vi "游标显示-步响应.vi"(3 "步响应计算参数 in":T2, 4 "试验模式":string, 5 "reference in":refnum<vi>) -> (0 "步响应计算参数 out":T2, 1 "试验模式 out":string, 2 "reference out":refnum<vi>)   [LabVIEW 2013]
panel:
  in  "Array":string[](array[string])=["行程", "油压1"]
  out "Yrange":dbl
  out "Xrange":dbl
  in  "Cursor":T1
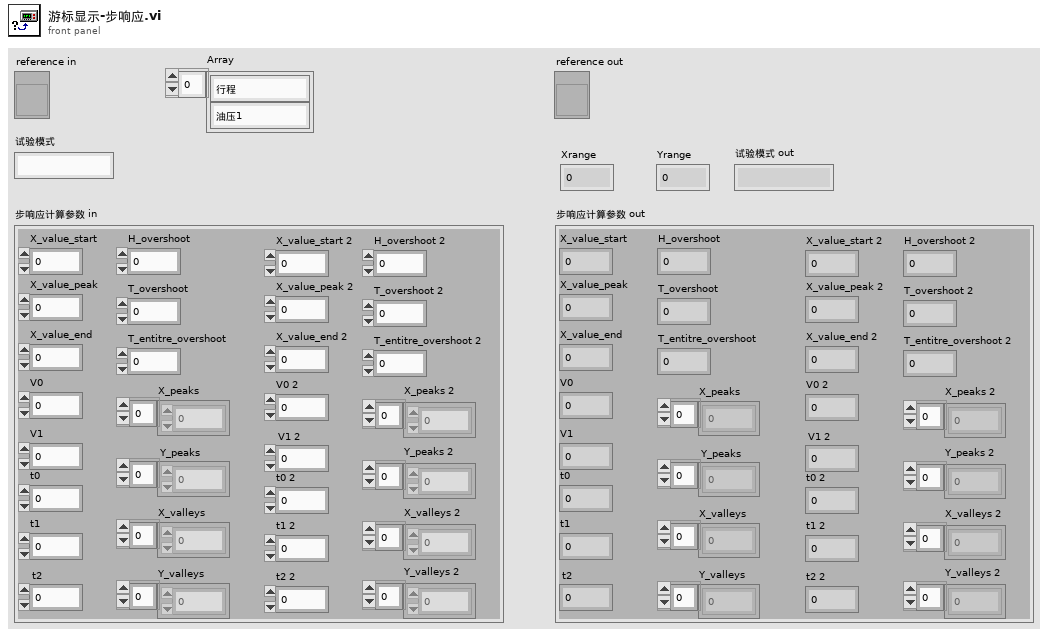
[diagram p1: front panel]
types:
  T1 = cluster{"Name":string, "Color":u32, "Style":u8, "Point Style":u8, "Name Visible":bool, "Allow Drag":bool, "Cursor Mode":u32, "Plot":i32, "Index":i32, "Position":cluster{"X":dbl, "Y":dbl}, "X Scale":u32, "Y Scale":u32, "Watch Plots":i32[], "Watch All Plots":bool, "Plot Area":i32, "Label Offset":cluster{"X":dbl, "Y":dbl}}
  T2 = cluster{"X_value_start":dbl, "X_value_peak":dbl, "t1":dbl, "X_value_end":dbl, "V0":dbl, "V1":dbl, "t0":dbl, "X_peaks":dbl[], "X_valleys":dbl[], "Y_peaks":dbl[], "Y_valleys":dbl[], "t2":dbl, "H_overshoot":dbl, "T_overshoot":dbl, "T_entitre_overshoot":dbl, "X_value_start 2":dbl, "X_value_peak 2":dbl, "t1 2":dbl, "X_value_end 2":dbl, "V0 2":dbl, "V1 2":dbl, "t0 2":dbl, "X_peaks 2":dbl[], "X_valleys 2":dbl[], "Y_peaks 2":dbl[], "t2 2":dbl, "H_overshoot 2":dbl, "T_overshoot 2":dbl, "T_entitre_overshoot 2":dbl, "Y_valleys 2":dbl[]}
  T3 = cluster{"Name":string, "Color":u32, "Style":u8, "Point Style":u8, "Name Visible":bool, "Allow Drag":bool, "Cursor Mode":u32, "Plot":i32, "Index":i32, "Position":cluster{"X":dbl, "Y":dbl}, "X Scale":u32, "Y Scale":u32, "Watch Plots":i32[], "Watch All Plots":bool, "Plot Area":i32, "Label Offset":cluster{"X":dbl, "Y":dbl}}[]
  T4 = typedef "LVCursorListTypeDef.ctl" = cluster{"Name":string, "Color":u32, "Style":u8, "Point Style":u8, "Name Visible":bool, "Allow Drag":bool, "Cursor Mode":u32, "Plot":i32, "Index":i32, "Position":cluster{"X":dbl, "Y":dbl}, "X Scale":u32, "Y Scale":u32, "Watch Plots":i32[], "Watch All Plots":bool, "Plot Area":i32, "Label Offset":cluster{"X":dbl, "Y":dbl}}[]
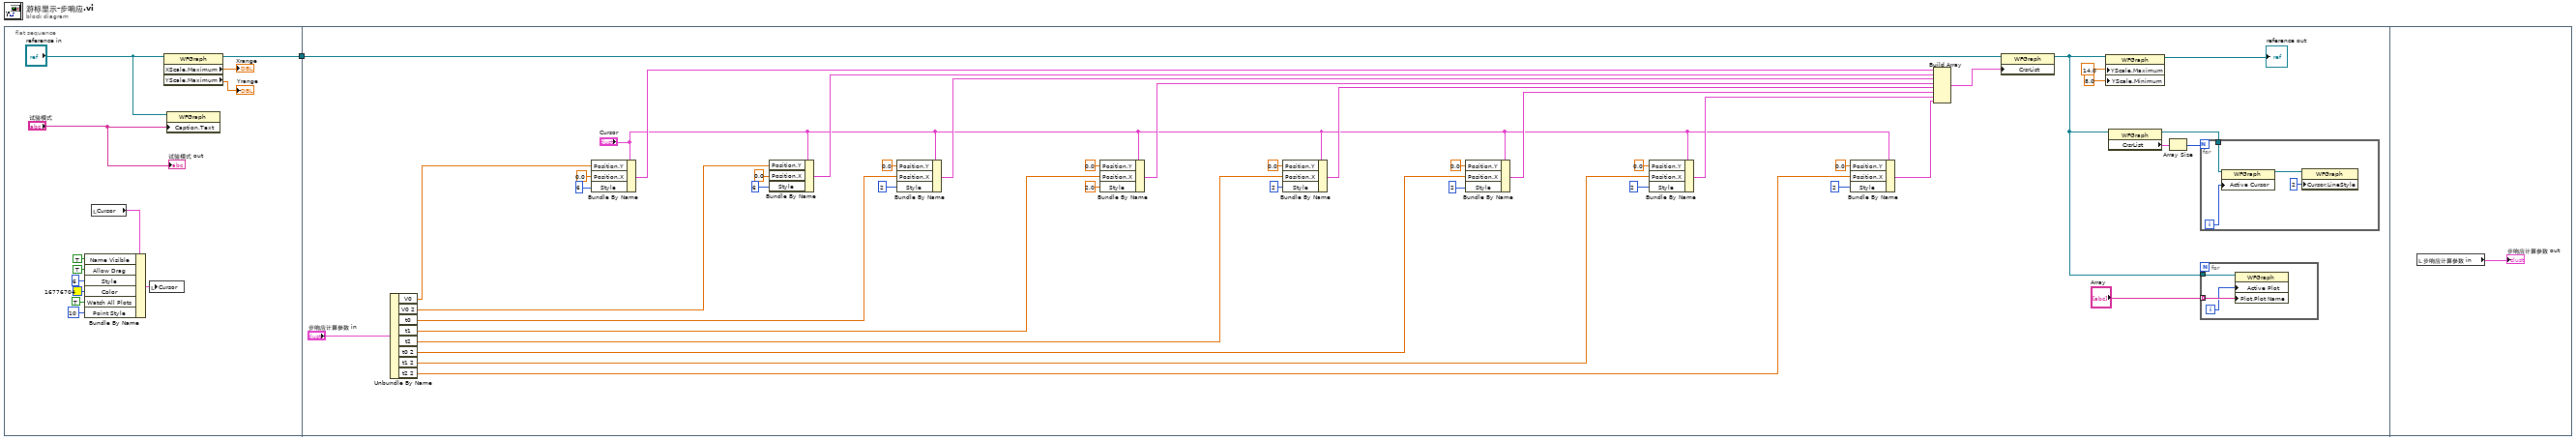
[diagram p0: block diagram]
diagram:
  n1 = flat-sequence {
    tunnel: [w4] -> w1
    tunnel: w1 -> [w47]
    frame #0 {
      n2 = local read "Cursor"() -> (w11:T1)
      n3 = Bundle By Name(cluster=w11, "Name Visible"=TRUE, "Allow Drag"=TRUE, "Style"=u8 6, "Color"=u32 16776704, "Watch All Plots"=TRUE, "Point Style"=u8 10) -> (w10:T1)
      n4 = local write "Cursor"(w10) -> ()
      n5 = property class="WFGraph"(reference="reference in") -> (reference out=w4:refnum<vi>, "XScale.Maximum"=→"Xrange":dbl, "YScale.Maximum"=→"Yrange":dbl)  [unwired: 1 in, 1 out]
      n6 = property on="Property Node" class="WFGraph"(reference="reference in", "Caption.Text"="试验模式") -> ()  [unwired: 1 in, 2 out]
      "试验模式 out" <- "试验模式"
    }
    frame #1 {
      n7 = Unbundle By Name("步响应计算参数 in") -> ("V0"=w37:dbl, "V0 2"=w36:dbl, "t0"=w32:dbl, "t1"=w31:dbl, "t2"=w29:dbl, "t0 2"=w28:dbl, "t1 2"=w26:dbl, "t2 2"=w25:dbl)
      n8 = Bundle By Name(cluster="Cursor", "Position.Y"=w37, "Position.X"=0.0, "Style"=u8 6) -> (w51:T1)
      n9 = Bundle By Name(cluster="Cursor", "Position.Y"=w36, "Position.X"=0.0, "Style"=u8 6) -> (w49:T1)
      n10 = Bundle By Name(cluster="Cursor", "Position.Y"=0.0, "Position.X"=w32, "Style"=u8 2) -> (w52:T1)
      n11 = Bundle By Name(cluster="Cursor", "Position.Y"=0.0, "Position.X"=w31, "Style"=2.0 ("Position.Y")) -> (w53:T1)
      n12 = Bundle By Name(cluster="Cursor", "Position.Y"=0.0, "Position.X"=w29, "Style"=u8 2) -> (w54:T1)
      n13 = Bundle By Name(cluster="Cursor", "Position.Y"=0.0, "Position.X"=w28, "Style"=u8 2) -> (w55:T1)
      n14 = Bundle By Name(cluster="Cursor", "Position.Y"=0.0, "Position.X"=w26, "Style"=u8 2) -> (w56:T1)
      n15 = Bundle By Name(cluster="Cursor", "Position.Y"=0.0, "Position.X"=w25, "Style"=u8 2) -> (w57:T1)
      n16 = Build Array(w51, w49, w52, w53, w54, w55, w56, w57) -> (w58:T3)
      n17 = property class="WFGraph"(reference=w47, "CrsrList"=w58) -> (reference out=w15:refnum<vi>)  [unwired: 1 in, 1 out]
      n18 = property on="属性节点" class="WFGraph"(reference=w15, "YScale.Maximum"=14.0 ("Y标尺.范围:最大值"), "YScale.Minimum"=8.0 ("Y标尺.范围:最小值")) -> (reference out=→"reference out":refnum<vi>)  [unwired: 1 in, 1 out]
      n19 = property class="WFGraph"(reference=w15) -> (reference out=w38:refnum<vi>, "CrsrList"=w40:T4)  [unwired: 1 in, 1 out]
      n20 = Array Size(array=w40) -> (size(s)=w39:i32)
      n21 = for {
        N: w39 -> [_]
        tunnel: w38 -> [w65]
        i -> [w64]
        n22 = property class="WFGraph"(reference=w65, "Active Cursor"=w64) -> (reference out=w63:refnum<vi>)  [unwired: 1 in, 1 out]
        n23 = property class="WFGraph"(reference=w63, "Cursor.LineStyle"=u8 2 ("Cursor.Line Style")) -> ()  [unwired: 1 in, 2 out]
      }
      n24 = for {
        tunnel: "Array" -> [w61] mode=indexing
        tunnel: w15 -> [w60]
        i -> [w59]
        n25 = property class="WFGraph"(reference=w60, "Active Plot"=w59, "Plot.Plot Name"=w61) -> ()  [unwired: 1 in, 2 out]
      }
    }
    frame #2 {
      n26 = local read "步响应计算参数 in"() -> (→"步响应计算参数 out":T2)
    }
  }
